vi "Update Info.vi"(8 "error in (no error)":errorcluster, 11 "Config Monitor Module in":refnum<class "Config Monitor Module.lvclass">) -> (0 "error out":errorcluster, 3 "Config Monitor Module out":refnum<class "Config Monitor Module.lvclass">, 4 "Node Config Info":T1[](array[typedef]))   [LabVIEW 2020, in "VolatusGUI.lvlib" / "Config Monitor Module.lvclass"]
uses:
  Config Monitor Module.lvclass
  C:/dev/lv20CE/relink/lv-volatus/Volatus/Module/Module.lvclass
  Node Config Info.ctl
  Config Monitor Module.lvclass/Config Monitor Module.ctl
  Module/Module.lvclass
  Volatus.lvlib
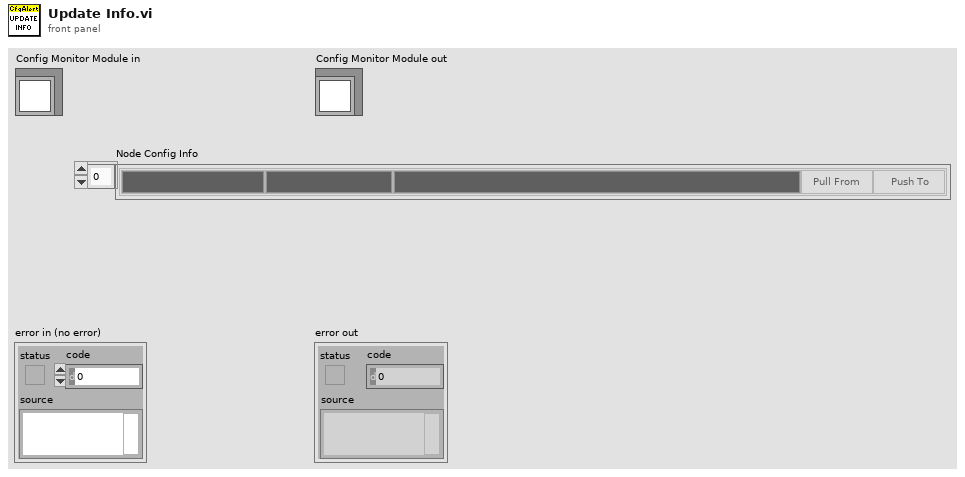
[diagram p1: front panel]
types:
  T1 = typedef "Volatus.lvlib/Node Config Info.ctl" = cluster{"Node":string, "Config Version":string, "Config Hash":string, "Pull":bool, "Push":bool, "Version Color":u32, "Hash Color":u32, "Node Color":u32}
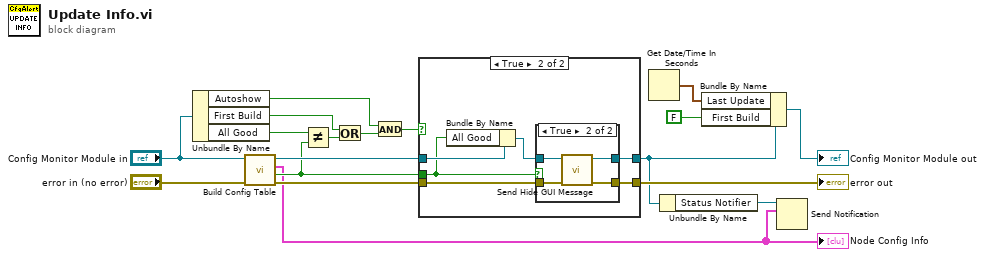
[diagram p0: block diagram]
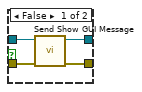
[diagram p3: hidden frame]
diagram:
  n1 = Unbundle By Name("Config Monitor Module in") -> ("Autoshow"=w9:bool, "First Build"=w12:bool, "All Good"=w18:bool)
  n2 = call "Build Config Table.vi"("error in (no error)"="error in (no error)", "Config Alert Module in"="Config Monitor Module in") -> ("error out"=w16:errorcluster, "All Good"=w14:bool, "Node Config Info"=w1:T1[], "Config Alert Module out"=w17:refnum<class "Config Monitor Module.lvclass">)  [unwired: 6 in]
  "Node Config Info" <- w1
  n3 = Not Equal?(x=w18, y=w14) -> (x != y?=w15:bool)
  n4 = Or(x=w12, y=w15) -> (x .or. y?=w13:bool)
  n5 = And(x=w9, y=w13) -> (x .and. y?=w10:bool)
  n6 = case shown="True" w10 {
    tunnel: w17 -> [w20 w26]
    tunnel: w16 -> [w19 w25]
    tunnel: w14 -> [_ w21]
    tunnel: [w20 w24] -> w3
    tunnel: [w19 w23] -> w5
    frame False {
    }
    frame True {
      n7 = Bundle By Name(cluster=w26, "All Good"=w21) -> (w22:refnum<class "Config Monitor Module.lvclass">)
      n8 = case shown="True" w21 {
        tunnel: w22 -> [w30 w32]
        tunnel: w25 -> [w29 w34]
        tunnel: [w28 w31] -> w24
        tunnel: [w27 w33] -> w23
        frame False {
          n9 = call "Send Show GUI Message.vi"("error in (no error)"=w29, "Module in"=w30) -> ("error out"=w27:errorcluster, "Module out"=w28:refnum<class "Config Monitor Module.lvclass">)  [unwired: 8 in]
        }
        frame True {
          n10 = call "Send Hide GUI Message.vi"("error in (no error)"=w34, "Module in"=w32) -> ("error out"=w33:errorcluster, "Module out"=w31:refnum<class "Config Monitor Module.lvclass">)  [unwired: 8 in]
        }
      }
    }
  }
  "error out" <- w5
  n11 = Get Date/Time In Seconds() -> (seconds since 1Jan1904=w6:timestamp)
  n12 = Unbundle By Name(w3) -> ("Status Notifier"=w2:refnum<notifier>)
  n13 = Bundle By Name(cluster=w3, "Last Update"=w6, "First Build"=FALSE) -> (→"Config Monitor Module out":refnum<class "Config Monitor Module.lvclass">)
  n14 = Send Notification(notification=w1, notifier=w2) -> ()  [unwired: 1 in, 2 out]
